vi "RSZVB Get Converter Power Offset.vi"(8 "error in (no error)":errorcluster {"code" format="%.0x"}, 9 "Port (1)":i32=1, 10 "Channel (1)":i32=1, 11 "VISA session":refnum<visa-resource-name>) -> (0 "error out":errorcluster {"code" format="%.0x"}, 1 "Port Power Offset":dbl format="%^.3e", 3 "dup VISA session":refnum<visa-resource-name>, 5 "Offset Parameter":i32)   [LabVIEW 2011]
doc: "This VI returns a source power or a power offset relative to the channel power for a frequency converter port <Pt>. An additional Cal Power Offset can be defined via SOURce<Ch>:POWer<Pt>:CORRection:LEVel:OFFSet. \n\nNotes:\n\n(1) This command is available for frequency converters with electronic attenuators R&S ZVA-ZxxxE.\n\nRemote-control command(s):\nSOURce<Ch>:POWer<Pt>:CONVerter:OFFSet?"
uses:
  _utility/RSZVB Global Data.vi
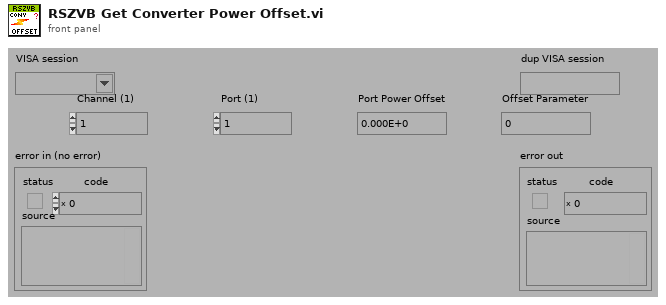
[diagram p1: front panel]
types:
  T1 = cluster{"Error Checking (T: On)":bool, "Installed Options":string[], "Data Valid?":bool, "Ports":i32, "Model":string[], "Option Checking (T: On)":bool}[]
  T2 = cluster{"Error Checking (T: On)":bool, "Installed Options":string[], "Data Valid?":bool, "Ports":i32, "Model":string[], "Option Checking (T: On)":bool}
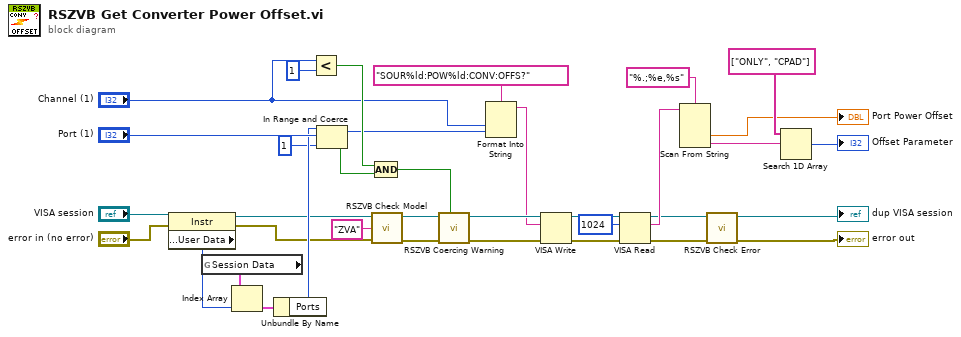
[diagram p0: block diagram]
diagram:
  n1 = property class="Instr"(reference="VISA session", error in="error in (no error)") -> (reference out=w23:refnum<visa-resource-name>, error out=w24:errorcluster, "General Settings:User Data"=w33:u32)
  n2 = global read "RSZVB Global Data.vi" "Session Data"() -> (w34:T1)
  n3 = Index Array(array=w34, index=w33) -> (element=w35:T2)
  n4 = Unbundle By Name(w35) -> ("Ports"=w29:i32)
  n5 = Less?(x="Channel (1)", y=1) -> (x < y?=w25:bool)
  n6 = In Range and Coerce(upper limit=w29, x="Port (1)", lower limit=1) -> (coerced(x)=w17:i32, In Range?=w26:bool)
  n7 = call "RSZVB Check Model.vi"("error in (no error)"=w24, "Model"="ZVA", "VISA session"=w23) -> ("error out"=w22:errorcluster, "dup VISA session"=w21:refnum<visa-resource-name>)  [unwired: 7 in]
  n8 = Compound Arithmetic op=AND(w25, w26) -> (w20:bool)
  n9 = call "RSZVB Coercing Warning.vi"("In Range?"=w20, "error in (no error)"=w22, "VISA session"=w21) -> ("error out"=w16:errorcluster, "dup VISA session"=w15:refnum<visa-resource-name>)  [unwired: 7 in]
  n10 = Format Into String(format string="SOUR%ld:POW%ld:CONV:OFFS?", "Channel (1)", w17) -> (resulting string=w14:string)  [unwired: 2 in, 1 out]
  n11 = VISA Write(VISA resource name=w15, write buffer=w14, error in (no error)=w16) -> (VISA resource name out=w12:refnum<visa-resource-name>, error out=w13:errorcluster)  [unwired: 1 out]
  n12 = VISA Read(VISA resource name=w12, byte count=u32 1024, error in (no error)=w13) -> (VISA resource name out=w7:refnum<visa-resource-name>, read buffer=w10:string, error out=w8:errorcluster)  [unwired: 1 out]
  n13 = Scan From String(format string="%.;%e,%s", input string=w10) -> (output 1=→"Port Power Offset":dbl, output 2=w6:string)  [unwired: 4 in, 3 out]
  n14 = call "RSZVB Check Error.vi"("error in (no error)"=w8, "VISA session"=w7) -> ("error out"=→"error out":errorcluster, "dup VISA session"=→"dup VISA session":refnum<visa-resource-name>)  [unwired: 8 in]
  n15 = Search 1D Array(1D array=string[] ["ONLY", "CPAD"], element=w6) -> (index of element=→"Offset Parameter":i32)  [unwired: 1 in]
